vi "Teleop with motor timer.vi"(10 "Match Info":T1={"Autonomous Elapsed Seconds"=0.0, "TeleOp Elapsed Seconds"=0.0, "Disabled Elapsed Seconds"=0.0, "Visited Autonomous"=FALSE, "Visited TeleOp"=FALSE, "Visited Disabled"=FALSE, "Autonomous Settings"={"Autonomous Style"=enum."Independent", "VI Refnum"=refnum}}, 11 "Call Context":T2) -> ()   [LabVIEW 2017]
doc: "This VI is called for each TeleOp packet received from the DS where the robot is not disabled. It is often used to read from the joysticks and update I/O or to update setpoints for timed control loops. It should complete and return within 20 milliseconds or it may miss DS packets."
uses:
  <vilib>/Rock Robotics/WPI/DriverStation/WPI_DriverStationDerivedRobotMode.ctl
  <vilib>/Rock Robotics/WPI/DriverStation/WPI_DriverStationMatch Info.ctl
  <vilib>/Rock Robotics/WPI/Utilities/WPI_GetSetVariantRefNum.vi
  <vilib>/Rock Robotics/Network Tables/NT Read Boolean.vi
  <vilib>/Rock Robotics/Network Tables/NT Read Number.vi
  <vilib>/Rock Robotics/Network Tables/NT Write Numeric Array.vi
panel:
  out "Sample Slider 0":dbl(slide) scale=0.0..5.0
  out "Sample Boolean 1":bool
  out "Sample Boolean 0":bool
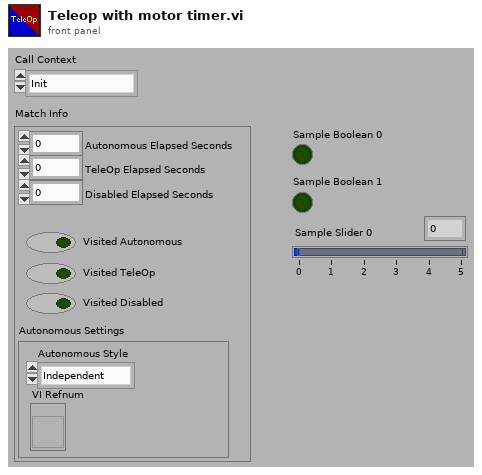
[diagram p1: front panel]
types:
  T1 = typedef "WPI_DriverStationMatch Info.ctl" = cluster{"Autonomous Elapsed Seconds":dbl, "TeleOp Elapsed Seconds":dbl, "Disabled Elapsed Seconds":dbl, "Visited Autonomous":bool, "Visited TeleOp":bool, "Visited Disabled":bool, "Autonomous Settings":cluster{"Autonomous Style":enum16{"Iterative", "Independent"}, "VI Refnum":refnum<vi>}}
  T2 = typedef "WPI_DriverStationDerivedRobotMode.ctl" = enum16{"Init", "Execute", "Stop"}
  T3 = typedef "WPI_JoystickDevRef.ctl" = cluster{"Device":T4}
  T4 = typedef "WPI_JoystickDeviceEnum.ctl" = enum16{"USB 0", "USB 1", "USB 2", "USB 3", "USB 4", "USB 5"}
  T5 = typedef "WPI_RobotDriveDevRef.ctl" = cluster{"DevStatus":errorcluster, "Motors[]":T6[], "Square Inputs":bool, "Max Output":dbl}
  T6 = typedef "WPI_MotorControlDeviceRef.ctl" = cluster{"DeviceStatus":errorcluster, "Type":T7, "PWM":cluster{"PWM Channel":T8, "DeadBand":T9}, "CAN":cluster{"Device Number":u8, "SetOutput VI Ref":variant, "GetOutput VI Ref":variant, "Enable VI Ref":variant, "Disable VI Ref":variant, "Data":variant}, "Invert":bool, "DIO PWM":cluster{"PWM \"Enable\" Channel":T8, "DIOChannel":T10, "PWM Rate":dbl}}
  T7 = typedef "WPI_MotorControlType.ctl" = enum16{"PWM", "CAN", "DIO PWM"}
  T8 = typedef "FPGA_DIOPWMChannel.ctl" = enum8{"PWM 0", "PWM 1", "PWM 2", "PWM 3", "PWM 4", "PWM 5", "PWM 6", "PWM 7", "PWM 8", "PWM 9", "PWM MXP 0", "PWM MXP 1", "PWM MXP 2", "PWM MXP 3", "PWM MXP 4", "PWM MXP 5", "PWM MXP 6", "PWM MXP 7", "PWM MXP 8", "PWM MXP 9", "Invalid"}
  T9 = typedef "WPI_PWMDeadband.ctl" = cluster{"Name":string, "maxPositivePwm":i32, "minPositivePwm":i32, "centerPwm":i32, "maxNegativePwm":i32, "minNegativePwm":i32, "angularRange":u16}
  T10 = typedef "FPGA_DIOChannel.ctl" = enum8{"DIO 0", "DIO 1", "DIO 2", "DIO 3", "DIO 4", "DIO 5", "DIO 6", "DIO 7", "DIO 8", "DIO 9", "DIO MXP 0", "DIO MXP 1", "DIO MXP 2", "DIO MXP 3", "DIO MXP 4", "DIO MXP 5", "DIO MXP 6", "DIO MXP 7", "DIO MXP 8", "DIO MXP 9", "DIO MXP 10", "DIO MXP 11", "DIO MXP 12", "DIO MXP 13", "DIO MXP 14", "DIO MXP 15", "SPI Port CS1", "SPI Port CS2", "SPI Port CS3", "SPI Port MISO", "SPI Port MOSI", "Invalid"}
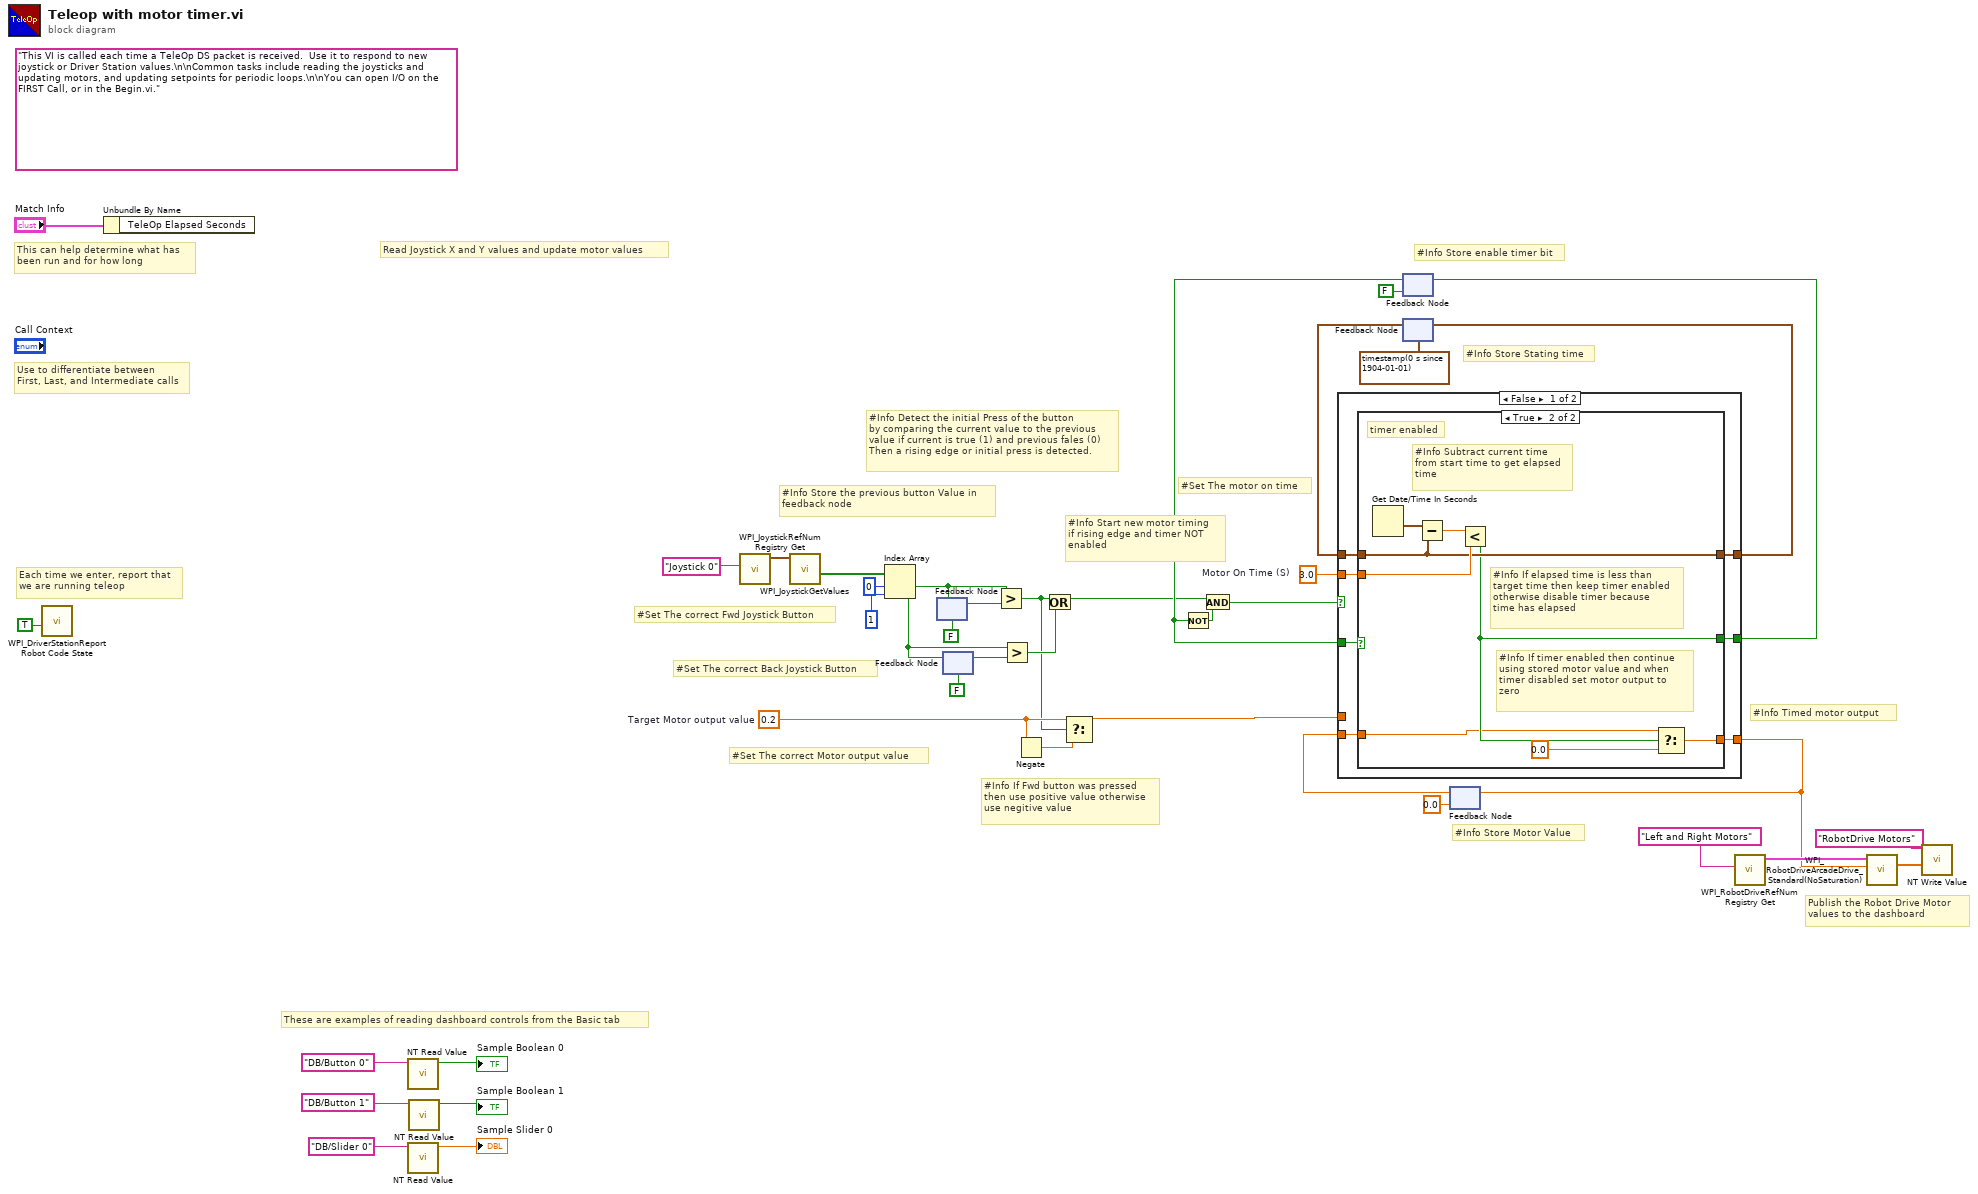
[diagram p0: block diagram]
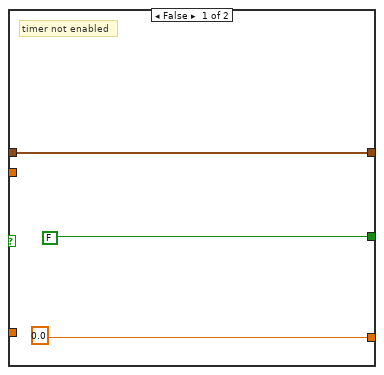
[diagram p2: hidden frame]
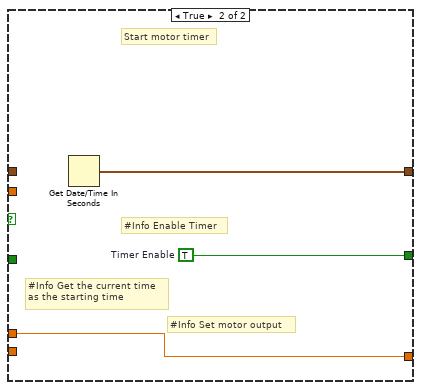
[diagram p3: hidden frame]
diagram:
  w3 = 0.2  # Target Motor output value
  w12 = 3.0  # Motor On Time (S)
  (unwired) "This VI is called each time a TeleOp DS packet is received.  Use it to respond to new joystick or Driver Station values.\n\nCommon tasks include reading the joysticks and updating motors, and updating setpoints for periodic loops.\n\nYou can open I/O on the FIRST Call, or in the Begin.vi."
  # "#Info If Fwd button was pressed\nthen use positive value otherwise\nuse negitive value"
  # "#Set The correct Back Joystick Button"
  # "#Info Timed motor output"
  # "#Set The correct Motor output value"
  # "#Set The motor on time"
  # "#Info Store Motor Value"
  # "#Info Start new motor timing\nif rising edge and timer NOT \nenabled"
  # "#Info Store enable timer bit"
  # "#Info Store Stating time"
  # "#Info Detect the initial Press of the button\nby comparing the current value to the previous\nvalue if current is true (1) and previous fales (0)\nThen a rising edge or initial press is detected."
  # "#Info Store the previous button Value in\nfeedback node"
  # "#Set The correct Fwd Joystick Button"
  # "These are examples of reading dashboard controls from the Basic tab"
  # "Publish the Robot Drive Motor\nvalues to the dashboard"
  # "Each time we enter, report that\nwe are running teleop"
  # "Use to differentiate between\nFirst, Last, and Intermediate calls"
  # "This can help determine what has\nbeen run and for how long"
  # "Read Joystick X and Y values and update motor values"
  n1 = call <vilib>:"WPI_DriverStationReport Robot Code State.vi"("TeleOp"=TRUE ("Autonomous")) -> ()  [unwired: 10 in, 1 out]
  n2 = Unbundle By Name("Match Info") -> ()  [unwired: 1 out]
  n3 = call-poly <vilib>:"NT Read Value.vi"("Name"="DB/Button 0" ("refnum name")) -> ("Boolean"=→"Sample Boolean 0":bool)  [unwired: 9 in, 1 out]
  n4 = call-poly <vilib>:"NT Read Value.vi"("Name"="DB/Slider 0" ("refnum name")) -> ("Numeric"=→"Sample Slider 0":dbl)  [unwired: 9 in, 1 out]
  n5 = call-poly <vilib>:"NT Read Value.vi"("Name"="DB/Button 1" ("refnum name")) -> ("Boolean"=→"Sample Boolean 1":bool)  [unwired: 9 in, 1 out]
  n6 = call <vilib>:"WPI_JoystickRefNum Registry Get.vi"("refnum name"="Joystick 0") -> ("JoystickDevRef"=w37:T3)  [unwired: 1 in, 9 out]
  n7 = call <vilib>:"WPI_JoystickGetValues.vi"("JoystickDevRef"=w37) -> ("Buttons"=w27:bool[])  [unwired: 6 in, 4 out]
  n8 = Index Array(array=w27, index #1=0 ("index"), index #2=1 ("index")) -> (element #1=w5:bool, element #2=w6:bool)
  n9 = feedback-in #1(w5) -> ()
  n10 = feedback #1(FALSE) -> (w25:bool)
  n11 = feedback #2(FALSE) -> (w8:bool)
  n12 = feedback-in #2(w6) -> ()
  n13 = Greater?(x=w5, y=w25) -> (0:w1:bool)
  n14 = Greater?(x=w6, y=w8) -> (0:w7:bool)
  n15 = Negate(x=w3) -> (-x=w2:dbl)
  n16 = Or(x=w1, y=w7) -> (x .or. y?=w10:bool)
  n17 = Select(t=w3, s=w1, f=w2) -> (s? t:f=w4:dbl)
  n18 = feedback #3(FALSE ("Timer Enable")) -> (w17:bool)
  n19 = Not(x=w17) -> (.not. x?=w16:bool)
  n20 = And(x=w10, y=w16) -> (x .and. y?=w18:bool)
  n21 = feedback #4(timestamp(0 s since 1904-01-01) ("seconds since 1Jan1904")) -> (w22:timestamp)
  n22 = feedback #5(0.0 ("upper limit")) -> (w14:dbl)
  n23 = case shown="False" w18 {
    tunnel: [w46 w62] -> w23
    tunnel: w22 -> [w47 _]
    tunnel: [w45 w61] -> w20
    tunnel: w17 -> [w48 _]
    tunnel: w4 -> [_ w60]
    tunnel: [w44 w60] -> w13
    tunnel: w14 -> [w42 _]
    tunnel: w12 -> [w43 _]
    frame False {
      n24 = case shown="True" w48 {
        tunnel: w47 -> [w51 w56]
        tunnel: [w51 w56] -> w46
        tunnel: [FALSE w55] -> w45
        tunnel: [0.0 ("upper limit") w52] -> w44
        tunnel: w43 -> [_ w57]
        tunnel: w42 -> [_ w54]
        frame False {
          # "timer not enabled"
        }
        frame True {
          # "#Info If timer enabled then continue\nusing stored motor value and when\ntimer disabled set motor output to\nzero"
          # "#Info If elapsed time is less than\ntarget time then keep timer enabled\notherwise disable timer because \ntime has elapsed"
          # "#Info Subtract current time\nfrom start time to get elapsed\ntime"
          # "timer enabled"
          n25 = Get Date/Time In Seconds() -> (seconds since 1Jan1904=w59:timestamp)
          n26 = Subtract(x=w59, y=w56) -> (x-y=w58:dbl)
          n27 = Less?(x=w58, y=w57) -> (x < y?=w55:bool)
          n28 = Select(t=w54, s=w55, f=0.0) -> (s? t:f=w52:dbl)
        }
      }
    }
    frame True {
      w61 = TRUE  # Timer Enable
      # "Start motor timer"
      # "#Info Set motor output"
      # "#Info Enable Timer"
      # "#Info Get the current time\nas the starting time"
      n29 = Get Date/Time In Seconds() -> (seconds since 1Jan1904=w62:timestamp)
    }
  }
  n30 = feedback-in #3(w20) -> ()
  n31 = feedback-in #4(w23) -> ()
  n32 = feedback-in #5(w13) -> ()
  n33 = call <vilib>:"WPI_RobotDriveRefNum Registry Get.vi"("refnum name"="Left and Right Motors") -> ("RobotDriveDevRef"=w39:T5)  [unwired: 1 in, 9 out]
  n34 = call <vilib>:"WPI_RobotDriveArcadeDrive_Standard(NoSaturation).vi"("X axis value"=w13, "RobotDriveDevRef"=w39) -> ("Motor Values"=w29:dbl[])  [unwired: 2 in, 7 out]
  n35 = call-poly <vilib>:"NT Write Value.vi"("Numeric Array"=w29, "Name"="RobotDrive Motors") -> ()  [unwired: 9 in, 1 out]
